vi "readmovement.vi"(0 "object in":refnum<class "Prior_Zmotor.lvclass">, 5 "error in (no error)":errorcluster) -> (14 "object out":refnum<class "Prior_Zmotor.lvclass">, 16 "IsMoving?":bool, 19 "error out":errorcluster)   [LabVIEW 2021, in "Prior_Zmotor.lvclass"]
uses:
  Prior_Zmotor.lvclass
  Prior_Zmotor.lvclass/Prior_Zmotor.ctl
panel:
  out "read buffer":string
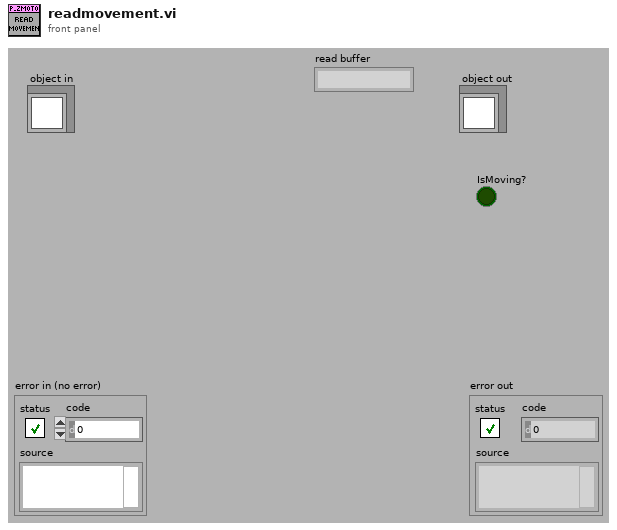
[diagram p1: front panel]
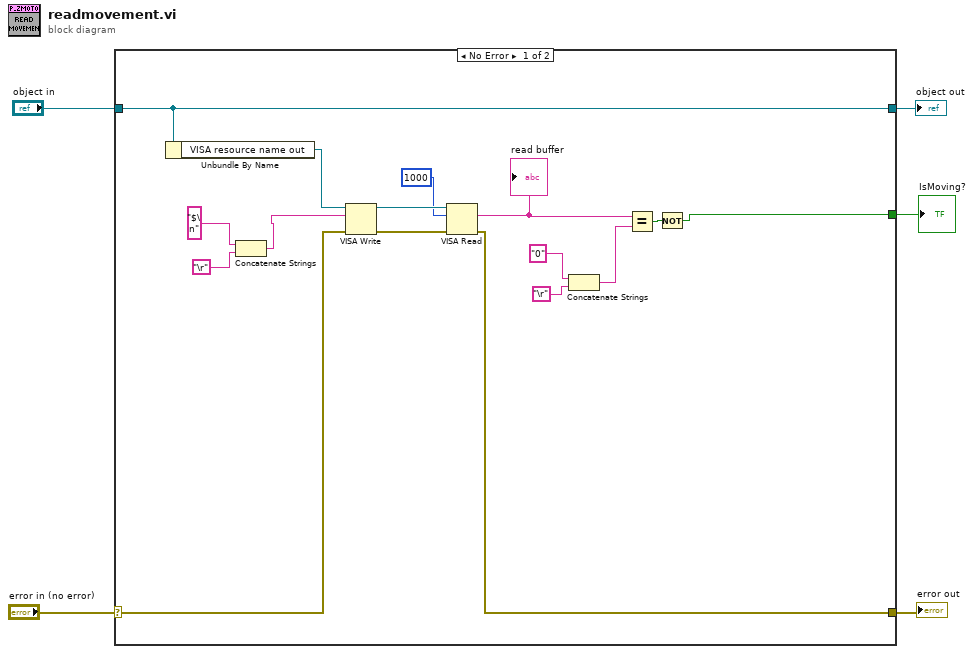
[diagram p0: block diagram]
diagram:
  n1 = case shown="No Error" "error in (no error)" {
    selector: "error in (no error)" -> [w19 w23]
    tunnel: [w16 w23] -> w4
    tunnel: [w21 w22] -> w2
    tunnel: "object in" -> [w21 w22]
    tunnel: [w13 _] -> w1
    frame No Error {
      n2 = Unbundle By Name(w21) -> ("VISA resource name out"=w20:refnum<visa-resource-name>)
      n3 = Concatenate Strings("$\n" ("write buffer"), "\r") -> (w9:string)
      n4 = VISA Write(VISA resource name=w20, write buffer=w9, error in (no error)=w19) -> (VISA resource name out=w18:refnum<visa-resource-name>, error out=w17:errorcluster)  [unwired: 1 out]
      n5 = VISA Read(VISA resource name=w18, byte count=u32 1000, error in (no error)=w17) -> (read buffer=w15:string, error out=w16:errorcluster)  [unwired: 2 out]
      "read buffer" <- w15
      n6 = Concatenate Strings("0" ("y"), "\r") -> (w6:string)
      n7 = Equal?(x=w15, y=w6) -> (x = y?=w14:bool)
      n8 = Not(x=w14) -> (.not. x?=w13:bool)
    }
    frame Error {
    }
  }
  "error out" <- w4
  "object out" <- w2
  "IsMoving?" <- w1
